vi "Main.vi"() -> ()   [LabVIEW 2019, in "HVC2.lvlib" / "HVC2.lvclass"]
uses:
  HVC2.lvclass
  typeDefs/Server State Data.ctl
  HVC2.lvclass/HVC2.ctl
panel:
  out "Numeric":i32
  out "error out":errorcluster
  in  "Stop":bool
  in  "Enable Async Mode":bool
  in  "Server Address":string="0.0.0.0:50051"
  in  "Server Certificate File (.crt)":path
  in  "Server Key File (.key)":path
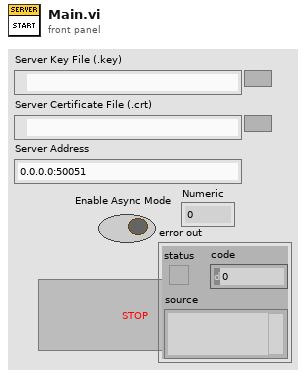
[diagram p1: front panel]
types:
  T1 = typedef "HVC2.lvlib/HVC2.lvclass/Server State Data.ctl" = cluster{"Data":string}
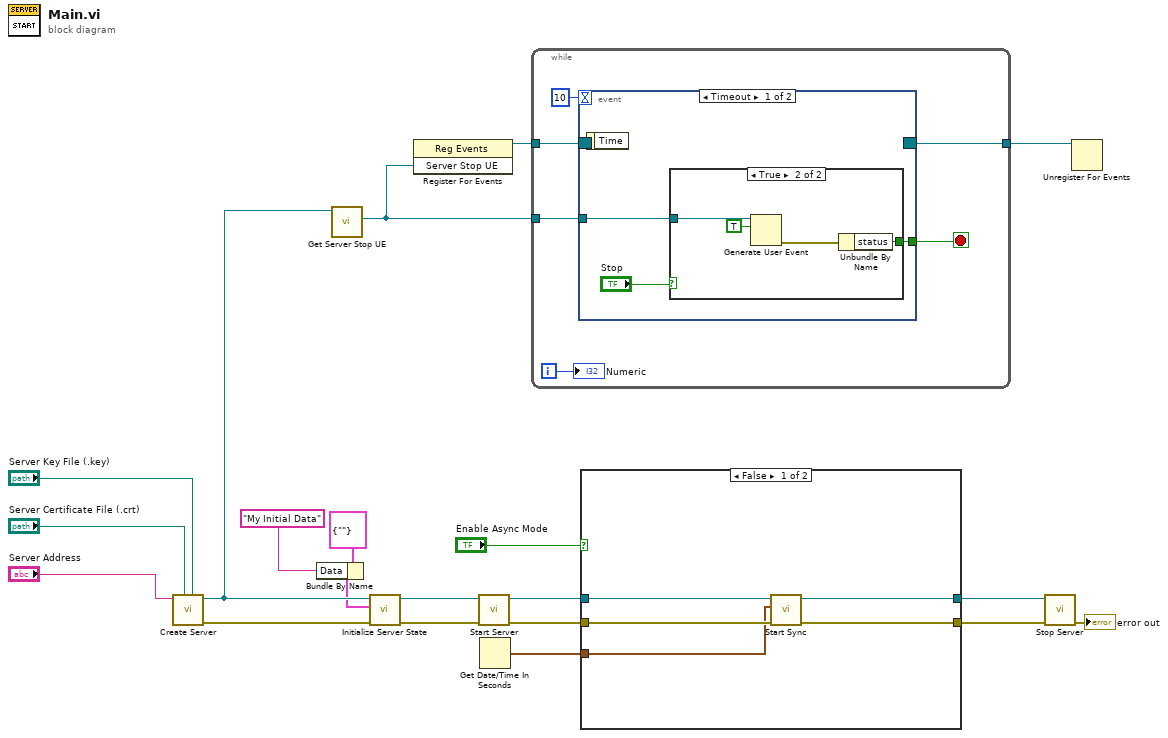
[diagram p0: block diagram]
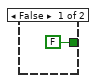
[diagram p2: hidden frame]
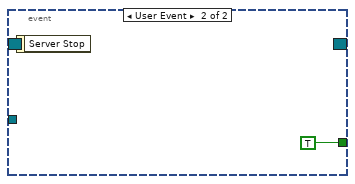
[diagram p3: hidden frame]
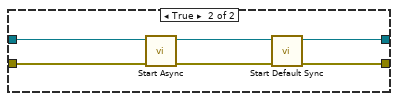
[diagram p4: hidden frame]
diagram:
  n1 = call "Create Server.vi"("Server Key File (.key)"="Server Key File (.key)", "Server Certificate File (.crt)"="Server Certificate File (.crt)", "Server Address"="Server Address") -> ("error out"=w9:errorcluster, "gRPC Server out"=w6:refnum<class "HVC2.lvclass">)  [unwired: 7 in]
  n2 = Bundle By Name(cluster=T1 {"Data"=""} ("Initial State"), "Data"="My Initial Data") -> (w4:T1)
  n3 = call "Get Server Stop UE.vi"("OOP Server in"=w6) -> ("Server Stop UE"=w10:refnum<user-event>)  [unwired: 9 in, 1 out]
  n4 = call "Initialize Server State.vi"("error in (no error)"=w9, "Initial State"=w4, "gRPC Server in"=w6) -> ("error out"=w8:errorcluster, "gRPC Server out"=w7:refnum<class "HVC2.lvclass">)  [unwired: 7 in]
  n5 = register-events(w10) -> (reference out=w12:refnum<event-registration>)  [unwired: 2 in, 1 out]
  n6 = call "Start Server.vi"("error in (no error)"=w8, "gRPC Server in"=w7) -> ("error out"=w20:errorcluster, "gRPC Server out"=w19:refnum<class "HVC2.lvclass">)  [unwired: 8 in]
  n7 = Get Date/Time In Seconds() -> (seconds since 1Jan1904=w2:timestamp)
  n8 = while {
    tunnel: w10 -> [w26]
    tunnel: w12 -> [w25]
    tunnel: [w23] -> w11
    i -> [w22]
    stop <- w24 stop-if-true
    n9 = event shown="[0] Timeout" {
      selector: w25 -> [_ _]
      dyn-events: [_ _] -> w23
      timeout: 10 -> [_ _]
      tunnel: w26 -> [w28 _]
      tunnel: [w29 TRUE] -> w24
      event Timeout {
        n10 = event-data() -> ()  [unwired: 1 in, 1 out]
        n11 = case shown="True" "Stop" {
          tunnel: [FALSE ("status") w32] -> w29
          tunnel: w28 -> [_ w31]
          frame False {
          }
          frame True {
            n12 = Generate User Event(user event=w31, event data cluster=TRUE ("event data")) -> (error out=w33:errorcluster)  [unwired: 2 in, 1 out]
            n13 = Unbundle By Name(w33) -> ("status"=w32:bool)
          }
        }
      }
      event User Event {
        n14 = event-data() -> ()  [unwired: 1 in, 1 out]
      }
    }
    "Numeric" <- w22
  }
  n15 = case shown="False" "Enable Async Mode" {
    tunnel: w20 -> [w40 w46]
    tunnel: w19 -> [w39 w45]
    tunnel: [w38 w42] -> w18
    tunnel: [w37 w41] -> w17
    tunnel: w2 -> [w36 _]
    frame False {
      n16 = call "Start Sync.vi"("error in (no error)"=w40, "current time"=w36, "gRPC Server in"=w39) -> ("error out"=w38:errorcluster, "gRPC Server out"=w37:refnum<class "HVC2.lvclass">)  [unwired: 7 in]
    }
    frame True {
      n17 = call "Start Async.vi"("error in (no error)"=w46, "gRPC Server in"=w45) -> ("error out"=w43:errorcluster, "gRPC Server out"=w44:refnum<class "HVC2.lvclass">)  [unwired: 8 in]
      n18 = call "Start Default Sync.vi"("error in (no error)"=w43, "gRPC Server in"=w44) -> ("error out"=w42:errorcluster, "gRPC Server out"=w41:refnum<class "HVC2.lvclass">)  [unwired: 8 in]
    }
  }
  n19 = call "Stop Server.vi"("error in (no error)"=w18, "gRPC Server in"=w17) -> ("error out"=→"error out":errorcluster)  [unwired: 9 in]
  n20 = Unregister For Events(event registration refnum=w11) -> ()  [unwired: 1 in, 1 out]
